vi "ErrorHandling.Fglb.GetHw.vi"(8 "error in (no error)":errorcluster) -> (0 "error out":errorcluster, 1 "error?":bool, 2 "Errors":T1[](array[typedef]))   [LabVIEW 2013]
uses:
  CitTemplate/citTemplate.errData.ctl
  EventLog/EventLog.EventSource.ctl
  ErrorHandling.Fglb.Action.ctl
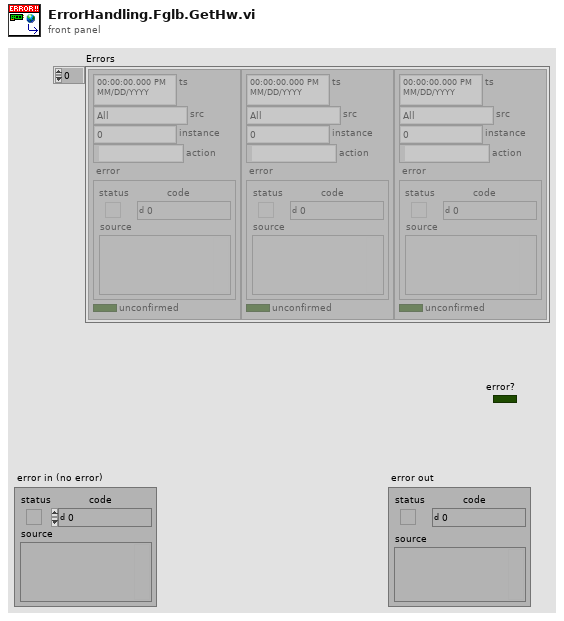
[diagram p1: front panel]
types:
  T1 = typedef "citTemplate.errData.ctl" = cluster{"ts":timestamp, "src":T2, "instance":i32, "action":string, "error":errorcluster, "unconfirmed":bool}
  T2 = typedef "EventLog.EventSource.ctl" = enum16{"All", "Gui", "Ref", "File", "Seq", "Scan", "AO", "AI", "DIO", "CPX", "M1", "M2", "DB"}
  T3 = typedef "ErrorHandling.Fglb.Action.ctl" = enum16{"init", "add", "clear", "confirm", "check", "get"}
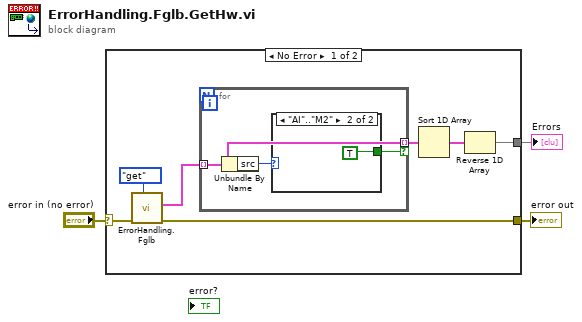
[diagram p0: block diagram]
diagram:
  n1 = case shown="No Error" "error in (no error)" {
    selector: "error in (no error)" -> [w8 w15]
    tunnel: [w9 w15] -> w3
    tunnel: [w4 _] -> w1
    frame No Error {
      n2 = call "ErrorHandling.Fglb.vi"("Action"=ErrorHandling.Fglb.Action."get", "error in (no error)"=w8) -> ("error out"=w9:errorcluster, "Errors out"=w6:T1[])  [unwired: 7 in, 1 out]
      n3 = for {
        tunnel: w6 -> [w13] mode=indexing
        tunnel: [w13] -> w7 mode=indexing if=w11
        n4 = Unbundle By Name(w13) -> ("src"=w12:T2)
        n5 = case shown="\"AI\"..\"M2\"" w12 {
          tunnel: [_ TRUE] -> w11
          frame Default {
          }
          frame "AI".."M2" {
          }
        }
      }
      n6 = Sort 1D Array(array=w7) -> (sorted array=w5:T1[])
      n7 = Reverse 1D Array(array=w5) -> (reversed array=w4:T1[])
    }
    frame Error {
    }
  }
  "error out" <- w3
  "Errors" <- w1
